vi "Init.vi"(0 "reference in":refnum<class "DAQ_Base.lvclass">, 5 "error in (no error)":errorcluster) -> (14 "reference out":refnum<class "DAQ_Base.lvclass">, 19 "error out":errorcluster)   [LabVIEW 2020, in "DAQ.lvlib" / "DAQ_Base.lvclass"]
uses:
  DAQ_Base.lvclass
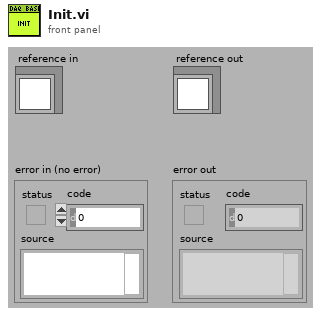
[diagram p1: front panel]
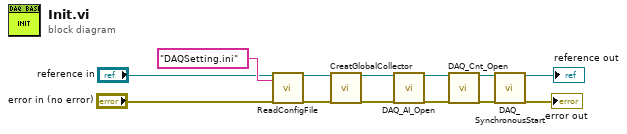
[diagram p0: block diagram]
diagram:
  n1 = call-dynamic "ReadConfigFile.vi"("reference in"="reference in", "ConfigFlieName"="DAQSetting.ini", "error in (no error)"="error in (no error)") -> ("reference out"=w10:refnum<class "DAQ_Base.lvclass">, "error out"=w9:errorcluster)  [unwired: 15 in]
  n2 = call-dynamic "CreatGlobalCollector.vi"("reference in"=w10, "error in (no error)"=w9) -> ("reference out"=w8:refnum<class "DAQ_Base.lvclass">, "error out"=w7:errorcluster)  [unwired: 16 in]
  n3 = call-dynamic "DAQ_AI_Open.vi"("reference in"=w8, "error in (no error)"=w7) -> ("reference out"=w6:refnum<class "DAQ_Base.lvclass">, "error out"=w5:errorcluster)  [unwired: 16 in]
  n4 = call-dynamic "DAQ_Cnt_Open.vi"("reference in"=w6, "error in (no error)"=w5) -> ("reference out"=w4:refnum<class "DAQ_Base.lvclass">, "error out"=w3:errorcluster)  [unwired: 16 in]
  n5 = call-dynamic "DAQ_SynchronousStart.vi"("reference in"=w4, "error in (no error)"=w3) -> ("reference out"=→"reference out":refnum<class "DAQ_Base.lvclass">, "error out"=→"error out":errorcluster)  [unwired: 16 in]
